vi "addTxBuffer.vi"(8 "error in (no error)":errorcluster, 10 "Frame":T1 {"Data" format="%02x"}, 11 "DesktopModbus in":refnum<class "DesktopModbus.lvclass">) -> (0 "error out":errorcluster, 3 "DesktopModbus out":refnum<class "DesktopModbus.lvclass">)   [LabVIEW 2015, in "DesktopModbus.lvclass"]
uses:
  DesktopModbus.lvclass
  Common_RT_Modbus/DataTypes/Frame.ctl
  DesktopModbus.lvclass/DesktopModbus.ctl
  Common_RT_Modbus/RTModbus.lvlib
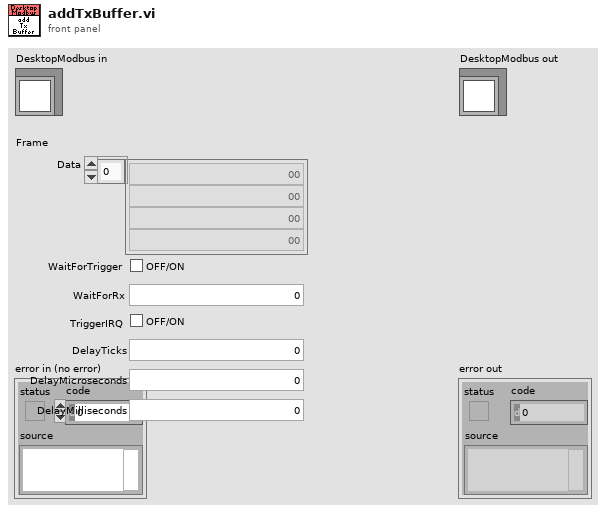
[diagram p1: front panel]
types:
  T1 = typedef "RTModbus.lvlib/Frame.ctl" = cluster{"Data":u8[], "WaitForTrigger":bool, "WaitForRx":u16, "TriggerIRQ":bool, "DelayTicks":u16, "DelayMicroseconds":u16, "DelayMilliseconds":u16}
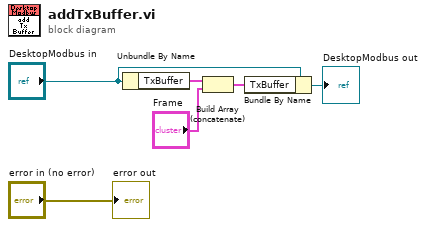
[diagram p0: block diagram]
diagram:
  n1 = Unbundle By Name("DesktopModbus in") -> ("TxBuffer"=w4:T1[])
  n2 = Build Array (concatenate)(w4, "Frame") -> (w2:T1[])
  n3 = Bundle By Name(cluster="DesktopModbus in", "TxBuffer"=w2) -> (→"DesktopModbus out":refnum<class "DesktopModbus.lvclass">)
  "error out" <- "error in (no error)"
